vi "Subsystem View.vi"(8 "error in (no error)":errorcluster, 10 "Subview Stop Event":refnum<user-event>, 11 "Subsystem URL":refnum<k21>) -> ()   [LabVIEW 2024]
doc: "Displays the graph of the specified subsystem and lists all I/O points in the subsystems. This VI is a subview of the Detailed View."
uses:
  Controls/Client/Alarm LED.ctl
  Controls/Client/Status LED.ctl
  Controls/Client/Subsystem View - Data.ctl
  Controls/Client/Initialization Status.ctl
  Shared/User Event - Stop.lvlib
  <vilib>/lvdsc/NI_DSC.lvlib
panel:
  out "Sampling Time dt (ms)":dbl
  out "In use?":T1
  out "error out":errorcluster
  out "Active Alarms?":T2
  out "Alarms?":T2
  in  "Set Point":dbl(slide) scale=0.0..100.0
  out "Process Value":dbl(slide) scale=0.0..100.0
  out "Integral":dbl
  out "Derivative":dbl
  out "Proportional":dbl
  out "Output":dbl(slide) scale=0.0..100.0
  out "Description":string
  in  "Variable List":i32(listbox)=1
  in  "Stop":bool
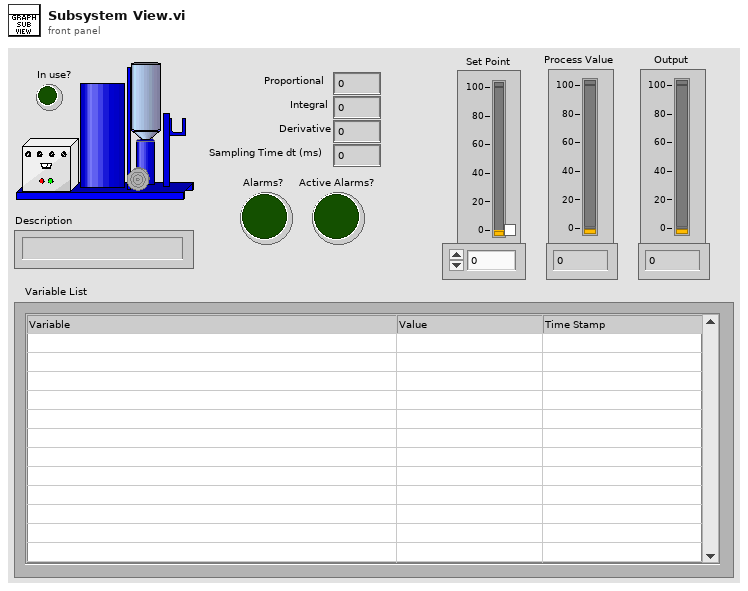
[diagram p1: front panel]
types:
  T1 = typedef "Status LED.ctl" = bool
  T2 = typedef "Alarm LED.ctl" = bool
  T3 = typedef "Subsystem View - Data.ctl" = cluster{"Subsystem URL":refnum<k21>, "Variables":refnum<k21>[], "URL Refnum Map":variant, "Subview Stop Event":refnum<user-event>, "Value Change Notifications":refnum<user-event>, "Initialization Status":T4, "Value List Reference":refnum<vi>}
  T4 = typedef "Initialization Status.ctl" = enum16{"Initializing", "Initialized"}
  T5 = cluster{"Min priority":u32, "Max priority":u32, "Show Acknowledged alarms?":bool}
  T6 = cluster{"# active alarms occurrences":i32, "any alarm occurrences?":bool, "# unack alarms occurrences":i32, "any unack alarm occurrences?":bool, "# shared variables with active alarms":i32, "any shared variables with alarms?":bool, "# shared variables with unack alarms":i32, "any shared variables with unack alarms?":bool}
  T7 = typedef "DEVT_Datatypes.ctl" = enum16{"No Value", "Custom", "Double", "Boolean", "U32", "String", "DBL Array", "I32 Array", "I32", "SGL Array", "SGL", "I8", "U8", "I16", "U16", "I64", "U64", "DBL Waveform", "I16 Waveform", "Boolean Array", "I8 Array", "U8 Array", "I16 Array", "U16 Array", "U32 Array", "I64 Array", "U64 Array", "DBL Waveform Array", "I16 Waveform Array"}
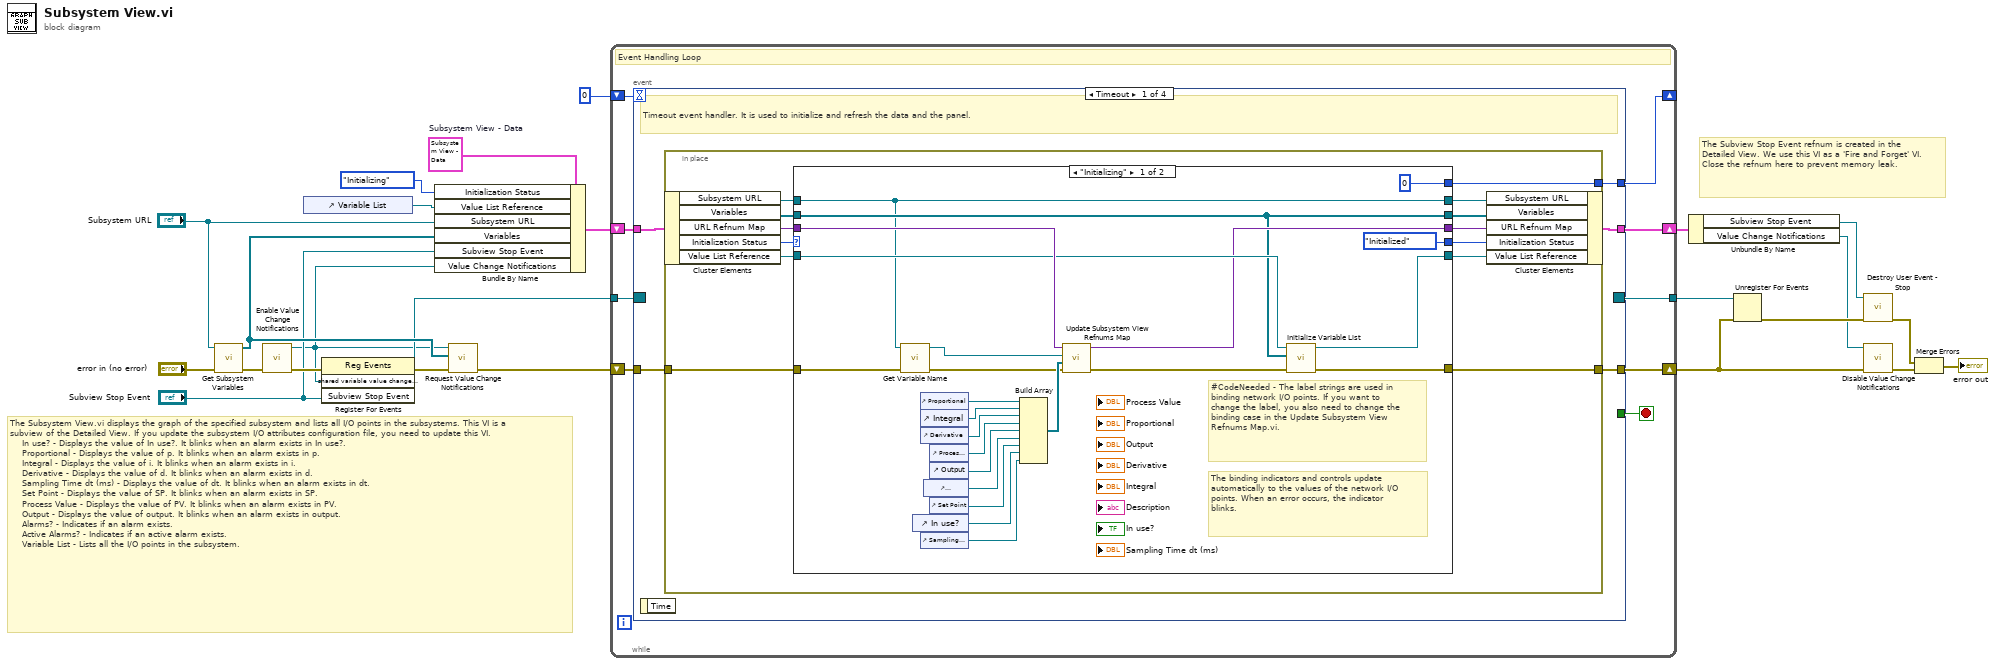
[diagram p0: block diagram]
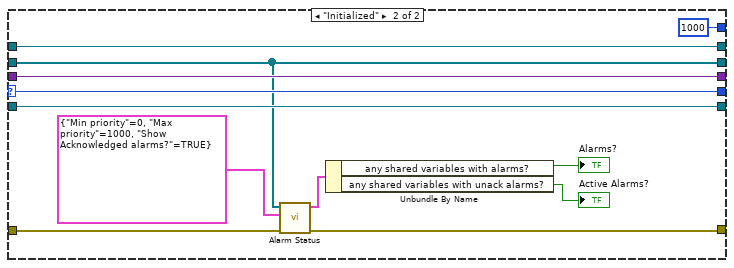
[diagram p2: hidden frame]
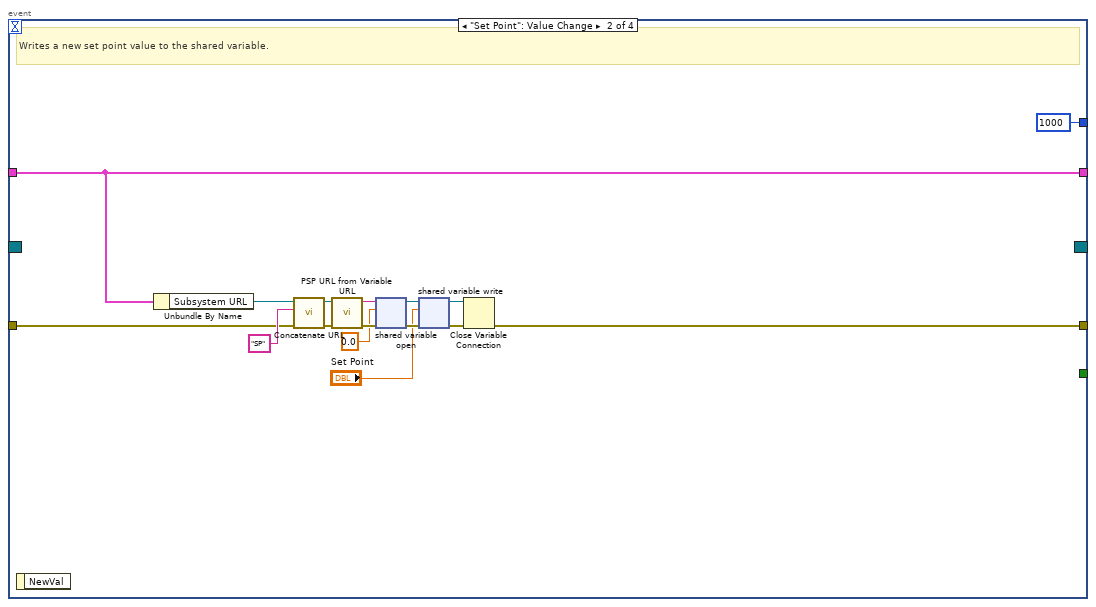
[diagram p3: hidden frame]
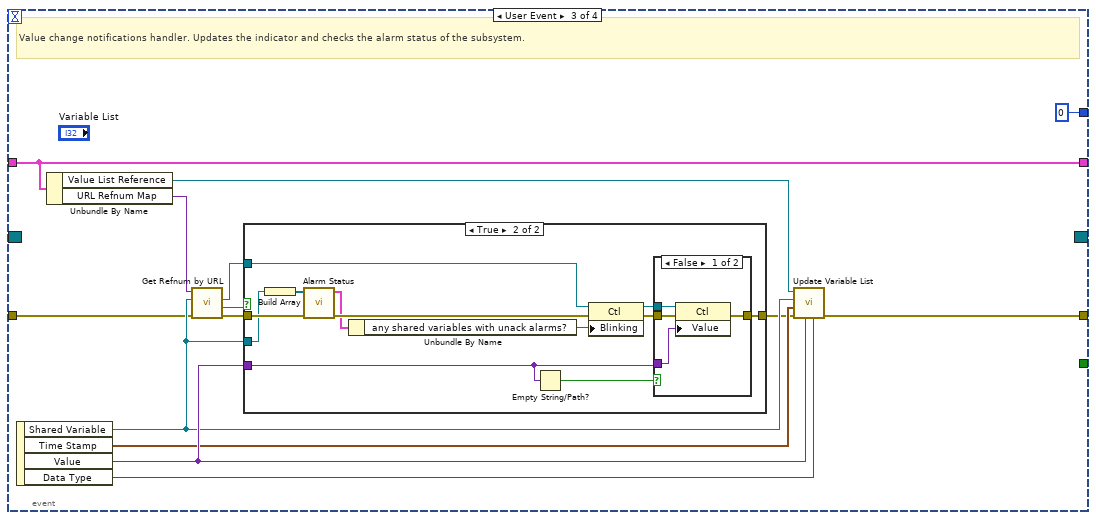
[diagram p4: hidden frame]
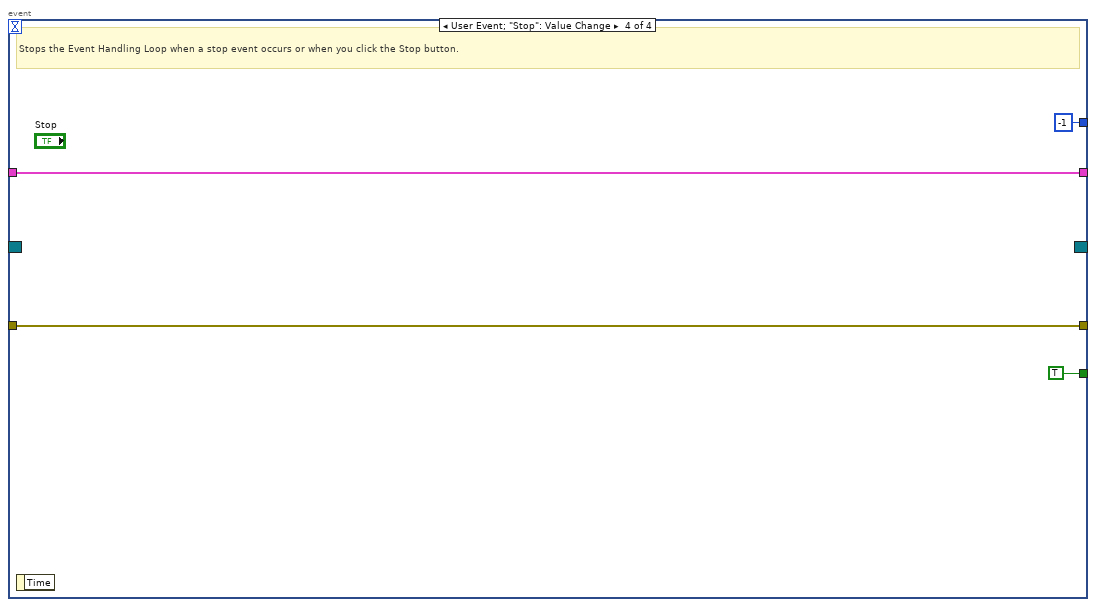
[diagram p7: hidden frame]
diagram:
  w12 = T3 {"Subsystem URL"="", "Variables"=[], "URL Refnum Map"=variant, "Subview Stop Event"=refnum, "Value Change Notifications"=refnum, "Initialization Status"=enum."Initializing", "Value List Reference"=refnum}  # Subsystem View - Data
  # "The Subview Stop Event refnum is created in the Detailed View. We use this VI as a 'Fire and Forget' VI. Close the refnum here to prevent memory leak."
  # "The Subsystem View.vi displays the graph of the specified subsystem and lists all I/O points in the subsystems. This VI is a subview of the Detailed View. If you update the subsystem I/O attributes configuration file, you need to update this VI.\n    In use? - Displays the value of In use?. It blinks when an alarm exists in In use?.\n    Proportional - Displays the value of p. It blinks when an alarm exists in p.\n    Integral - Displays the value of i. It blinks when an alarm exists in i.\n    Derivative - Displays the value of d. It blinks when an alarm exists in d.\n    Sampling Time dt (ms) - Displays the value of dt. It blinks when an alarm exists in dt.\n    Set Point - Displays the value of SP. It blinks when an alarm exists in SP.\n    Process Value - Displays the value of PV. It blinks when an alarm exists in PV.\n    Output - Displays the value of output. It blinks when an alarm exists in output.\n    Alarms? - Indicates if an alarm exists.\n    Active Alarms? - Indicates if an active alarm exists.\n    Variable List - Lists all the I/O points in the subsystem."
  n1 = call "Get Subsystem Variables.vi"("error in (no error)"="error in (no error)", "Subsystem URL"="Subsystem URL") -> ("error out"=w17:errorcluster, "Variable URLs"=w24:refnum<k21>[])  [unwired: 6 in, 2 out]
  n2 = call <vilib>:"Enable Value Change Notifications.vi"("error in (no error)"=w17) -> ("error out"=w18:errorcluster, "shared variable value change notification"=w5:refnum<user-event>)  [unwired: 9 out]
  n3 = control-ref of="Variable List"() -> (w3:refnum<vi>)
  n4 = register-events(error in=w18, w5, "Subview Stop Event") -> (reference out=w22:refnum<event-registration>, error out=w23:errorcluster)  [unwired: 1 in]
  n5 = Bundle By Name(cluster=w12, "Initialization Status"=enum16{"Initializing", "Initialized"}."Initializing", "Value List Reference"=w3, "Subsystem URL"="Subsystem URL", "Variables"=w24, "Subview Stop Event"="Subview Stop Event", "Value Change Notifications"=w5) -> (w7:T3)
  n6 = call <vilib>:"Request Value Change Notifications.vi"("error in (no error)"=w23, "shared variables"=w24, "notification refnum"=w5) -> ("error out"=w21:errorcluster)  [unwired: 1 in, 7 out]
  n7 = while {
    shift-right: [w30] -> w16
    shift-left: w21 -> [w31]
    tunnel: w22 -> [w32]
    tunnel: [w29] -> w20
    shift-right: [w25] -> _
    shift-left: 0 -> [w28]
    shift-right: [w26] -> w10
    shift-left: w7 -> [w27]
    stop <- w33 stop-if-true
    # "Event Handling Loop"
    n8 = event shown="[0] Timeout" {
      selector: w32 -> [_ _ _ _]
      dyn-events: [_ _ _ _] -> w29
      timeout: w28 -> [_ _ _ _]
      tunnel: [_ _ _ TRUE] -> w33
      tunnel: w31 -> [w35 w93 w108 w137]
      tunnel: [w36 w89 w113 w137] -> w30
      tunnel: w27 -> [w38 w92 w104 w135]
      tunnel: [w37 w92 w104 w135] -> w26
      tunnel: [w34 1000 0 -1] -> w25
      event Timeout {
        # "Timeout event handler. It is used to initialize and refresh the data and the panel."
        n9 = event-data() -> ()  [unwired: 1 in, 1 out]
        n10 = in-place {
          in-place-border: [w41] -> w36
          in-place-border: w35 -> [w40]
          in-place-border: [w39] -> w34
          n11 = in-place-cluster #1(w38) -> ("Subsystem URL"=w50:refnum<k21>, "Variables"=w48:refnum<k21>[], "URL Refnum Map"=w51:variant, "Initialization Status"=w49:T4, "Value List Reference"=w47:refnum<vi>)
          n12 = case shown="\"Initializing\"" w49 {
            selector: w49 -> [_ w85]
            tunnel: [w72 w75] -> w41
            tunnel: w50 -> [w57 w83]
            tunnel: w51 -> [w74 w84]
            tunnel: w40 -> [w56 w79]
            tunnel: w48 -> [w67 w78]
            tunnel: w47 -> [w71 w86]
            tunnel: [w70 w86] -> w46
            tunnel: [enum16{"Initializing", "Initialized"}."Initialized" ("Initialization Status") w85] -> w45
            tunnel: [w68 w84] -> w44
            tunnel: [w67 w78] -> w43
            tunnel: [w57 w83] -> w42
            tunnel: [0 1000] -> w39
            frame "Initializing" {
              # "#CodeNeeded - The label strings are used in binding network I/O points. If you want to change the label, you also need to change the binding case in the Update Subsystem View Refnums Map.vi."
              # "The binding indicators and controls update automatically to the values of the network I/O points. When an error occurs, the indicator blinks."
              n13 = call "Get Variable Name.vi"("error in (no error)"=w56, "Variable URL"=w57) -> ("error out"=w55:errorcluster, "dup Variable URL"=w54:refnum<k21>)  [unwired: 7 in, 1 out]
              n14 = control-ref of="In use?"() -> (w53:refnum<vi>)
              n15 = control-ref of="Proportional"() -> (w65:refnum<vi>)
              n16 = control-ref of="Integral"() -> (w64:refnum<vi>)
              n17 = control-ref of="Derivative"() -> (w63:refnum<vi>)
              n18 = control-ref of="Sampling Time dt (ms)"() -> (w52:refnum<vi>)
              n19 = control-ref of="Description"() -> (w66:refnum<vi>)
              n20 = control-ref of="Process Value"() -> (w62:refnum<vi>)
              n21 = control-ref of="Output"() -> (w61:refnum<vi>)
              n22 = control-ref of="Set Point"() -> (w58:refnum<vi>)
              n23 = Build Array(w65, w64, w63, w62, w61, w66, w58, w53, w52) -> (w60:refnum<vi>[])
              n24 = call "Update Subsystem View Refnums Map.vi"("error in (no error)"=w55, "Binding Control Refnums"=w60, "Subsystem URL"=w54, "URL Refnum Map In"=w74) -> ("error out"=w73:errorcluster, "URL Refnum Map Out"=w68:variant)  [unwired: 5 in, 1 out]
              n25 = call "Initialize Variable List.vi"("error in (no error)"=w73, "Variable URLs In"=w67, "Value List Reference In"=w71) -> ("error out"=w72:errorcluster, "Value List Reference Out"=w70:refnum<vi>)  [unwired: 6 in, 1 out]
            }
            frame "Initialized" {
              n26 = call <vilib>:"Alarm Status.vi"("error in (no error)"=w79, "read parameters"=T5 {"Min priority"=0, "Max priority"=1000, "Show Acknowledged alarms?"=TRUE}, "shared variables"=w78) -> ("error out"=w75:errorcluster, "alarm summary data"=w81:T6)  [unwired: 7 in]
              n27 = Unbundle By Name(w81) -> ("any shared variables with alarms?"=→"Alarms?":bool, "any shared variables with unack alarms?"=→"Active Alarms?":bool)
            }
          }
          n28 = in-place-cluster #1("Subsystem URL"=w42, "Variables"=w43, "URL Refnum Map"=w44, "Initialization Status"=w45, "Value List Reference"=w46) -> (w37:T3)
        }
      }
      event "Set Point": Value Change {
        # "Writes a new set point value to the shared variable."
        n29 = event-data() -> ()  [unwired: 1 in, 1 out]
        n30 = Unbundle By Name(w92) -> ("Subsystem URL"=w91:refnum<k21>)
        n31 = call "Concatenate URL.vi"("error in (no error)"=w93, "Child Name"="SP", "Parent URL"=w91) -> ("error out"=w95:errorcluster, "Child URL"=w97:refnum<k21>)  [unwired: 7 in]
        n32 = call "PSP URL from Variable URL.vi"("error in (no error)"=w95, "Shared Variable URL"=w97) -> ("error out"=w94:errorcluster, "PSP URL"=w96:string)  [unwired: 8 in]
        n33 = shared-variable-open(w96, w94, 0.0 ("New Value")) -> (w101:refnum<k21>, w100:errorcluster)  [unwired: 1 in]
        n34 = shared-variable-write(w101, w100, "Set Point") -> (w99:refnum<k21>, w98:errorcluster)
        n35 = Close Variable Connection(8:w98, 11:w99) -> (0:w89:errorcluster)
      }
      event User Event {
        # "Value change notifications handler. Updates the indicator and checks the alarm status of the subsystem."
        n36 = event-data() -> ("Shared Variable"=w109:refnum<k21>, "Time Stamp"=w110:timestamp, "Value"=w111:variant, "Data Type"=w112:T7)  [unwired: 1 in]
        n37 = Unbundle By Name(w104) -> ("Value List Reference"=w105:refnum<vi>, "URL Refnum Map"=w106:variant)
        n38 = call "Get Refnum by URL.vi"("error in (no error)"=w108, "URL"=w109, "Map In"=w106) -> ("error out"=w114:errorcluster, "Found?"=w116:bool, "Control Refnum"=w115:refnum<vi>)  [unwired: 5 in, 1 out]
        n39 = case shown="True" w116 {
          tunnel: w115 -> [_ w124]
          tunnel: w111 -> [_ w122]
          tunnel: w114 -> [w117 w128]
          tunnel: w109 -> [_ w121]
          tunnel: [w117 w123] -> w107
          frame False {
          }
          frame True {
            n40 = Build Array(w121) -> (w120:refnum<k21>[])
            n41 = call <vilib>:"Alarm Status.vi"("error in (no error)"=w128, "shared variables"=w120) -> ("error out"=w126:errorcluster, "alarm summary data"=w119:T6)  [unwired: 8 in]
            n42 = Unbundle By Name(w119) -> ("any shared variables with unack alarms?"=w118:bool)
            n43 = Empty String/Path?(string/path=w122) -> (empty?=w129:bool)
            n44 = property class="Ctl"(reference=w124, error in=w126, "Blinking"=w118) -> (reference out=w125:refnum<vi>, error out=w127:errorcluster)
            n45 = case shown="False" w129 {
              tunnel: w125 -> [w133 _]
              tunnel: w122 -> [w132 _]
              tunnel: w127 -> [w131 w134]
              tunnel: [w130 w134] -> w123
              frame False {
                n46 = property class="Ctl"(reference=w133, error in=w131, "Value"=w132) -> (error out=w130:errorcluster)  [unwired: 1 out]
              }
              frame True {
              }
            }
          }
        }
        n47 = call "Update Variable List.vi"("Data Type"=w112, "Value"=w111, "error in (no error)"=w107, "Time Stamp"=w110, "Shared Variable"=w109, "Value List Reference In"=w105) -> ("error out"=w113:errorcluster)  [unwired: 4 in, 1 out]
      }
      event User Event; "Stop": Value Change {
        # "Stops the Event Handling Loop when a stop event occurs or when you click the Stop button."
        n48 = event-data() -> ()  [unwired: 1 in, 1 out]
      }
    }
  }
  n49 = Unbundle By Name(w10) -> ("Subview Stop Event"=w9:refnum<user-event>, "Value Change Notifications"=w8:refnum<user-event>)
  n50 = Unregister For Events(event registration refnum=w20, error in=w16) -> (error out=w13:errorcluster)
  n51 = call "Destroy User Event - Stop.vi"("error in (no error)"=w13, "User Event - Stop"=w9) -> ("error out"=w15:errorcluster)  [unwired: 9 in]
  n52 = call <vilib>:"Disable Value Change Notifications.vi"("error in (no error)"=w16, "notification refnum"=w8) -> ("error out"=w19:errorcluster)  [unwired: 9 out]
  n53 = Merge Errors(w15, w19) -> (→"error out":errorcluster)
